vi "RSNRPZ Self-Test.vi"(8 "error in (no error)":errorcluster, 11 "VISA session":refnum<visa-resource-name> caption="VISA resource name") -> (0 "error out":errorcluster, 1 "Self-Test Message":string, 2 "Self Test Result":i16 format="%.0x", 3 "dup VISA session":refnum<visa-resource-name> caption="VISA resource name")   [LabVIEW 2010]
doc: "This VI runs the instrument's self test routine and returns the test result(s)."
uses:
  rsnrpz_32.dll
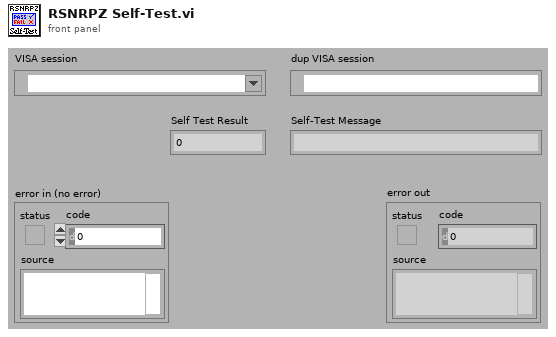
[diagram p1: front panel]
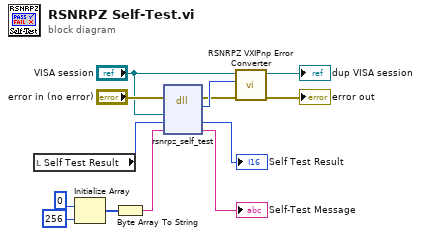
[diagram p0: block diagram]
diagram:
  n1 = local read "Self Test Result"() -> (w9:i16)
  n2 = Initialize Array(u8 0, 256) -> (w11:u8[])
  n3 = Byte Array To String(unsigned byte array=w11) -> (string=w7:string)
  n4 = dll-call lib="rsnrpz_32.dll" fn="rsnrpz_self_test"(error in="error in (no error)", "VISA Session"="VISA session", "Self Test Result"=w9, "Self-Test Message"=w7) -> (error out=w5:errorcluster, "Status"=w10:i32, "Self Test Result"=→"Self Test Result":i16, "Self-Test Message"=→"Self-Test Message":string)  [unwired: 3 in, 1 out]
  n5 = call <instrlib>:"RSNRPZ VXIPnp Error Converter.vi"("error in"=w5, "VXIPnp error code"=w10, "VISA session"="VISA session") -> ("error out"=→"error out":errorcluster, "dup VISA session"=→"dup VISA session":refnum<visa-resource-name>)  [unwired: 7 in]
